vi "Get AI REF StringsAndValues.vi"(8 "error in (no error)":errorcluster, 11 "Channels.REF":T1 {"Roll-Off" min=1; "TC" min=0.0001 format="%#_3p"; "Phase" format="%.3g"; "Frequency" min=0.0001 max=10000.0 format="%.3g"; "Channel" min=1}) -> (0 "error out":errorcluster, 2 "REF StringsAndValues":cluster{string, i32}[](array[cluster]))   [LabVIEW 2019, in "Instrument.Lockin.lvlib" / "Instrument UI.Lockin.lvclass"]
uses:
  Instrument UI.Lockin.lvclass
  Instrument.DAQ/Typedefs/REF.Channel--Cluster--Array.ctl
  Instrument.DAQ/Typedefs/REF.Channel--Cluster.ctl
  Instrument.DAQ/Instrument.DAQ.lvclass
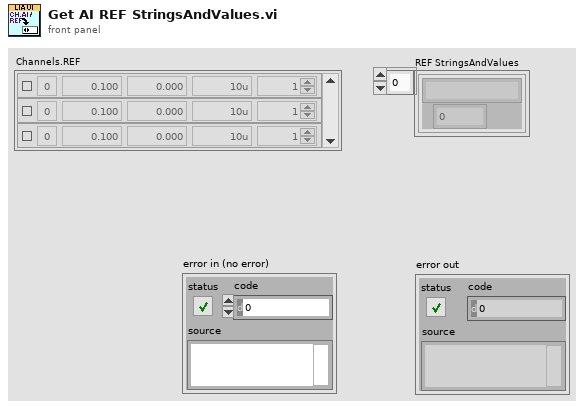
[diagram p1: front panel]
types:
  T1 = typedef "Instrument.Lockin.lvlib/Instrument.DAQ.lvclass/REF.Channel--Cluster--Array.ctl" = T2[]
  T2 = typedef "Instrument.Lockin.lvlib/Instrument.DAQ.lvclass/REF.Channel--Cluster.ctl" = cluster{"Enable?":bool, "Channel":i32, "Frequency":dbl, "Phase":dbl, "TC":dbl, "Roll-Off":i32}
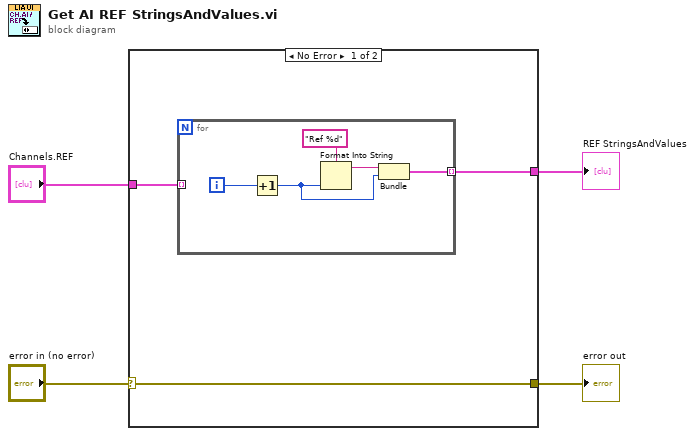
[diagram p0: block diagram]
diagram:
  n1 = case shown="No Error" "error in (no error)" {
    selector: "error in (no error)" -> [w6 w13]
    tunnel: [w7 _] -> w4
    tunnel: [w6 w13] -> w2
    tunnel: "Channels.REF" -> [w5 _]
    frame No Error {
      n2 = for {
        tunnel: [w12] -> w7 mode=indexing
        tunnel: w5 -> [_] mode=indexing
        i -> [w10]
        n3 = Increment(x=w10) -> (x+1=w8:i32)
        n4 = Format Into String(format string="Ref %d", w8) -> (resulting string=w9:string)  [unwired: 2 in, 1 out]
        n5 = Bundle(w9, w8) -> (w12:cluster{string, i32})  [unwired: 1 in]
      }
    }
    frame Error {
    }
  }
  "REF StringsAndValues" <- w4
  "error out" <- w2
